vi "DoStuff.vi"(0 "Subnet in":refnum<class "Subnet.lvclass">, 9 "Steps":i32) -> (4 "Subnet out":refnum<class "Subnet.lvclass">, 6 "BroadcastCounter":u8, 8 "ValidCRC":i32, 10 "InvalidCRC":i32, 13 "CRCIssues":T1[](array[typedef]) {"Data" format="%02x"}, 14 "Messages":i32, 15 "error out":errorcluster)   [LabVIEW 2016]
uses:
  Subnet/Subnet.lvclass
  Common_RT_Modbus/DataTypes/RxFrame.ctl
  Subnet/Subnet.lvclass/Subnet.ctl
  Common_RT_HPILC/HPILC/HPILC.lvclass/HPILC.ctl
  Common_RT_HPILC/HPILC/HPILC.lvclass
  Common_RT_Modbus/RTModbus.lvlib
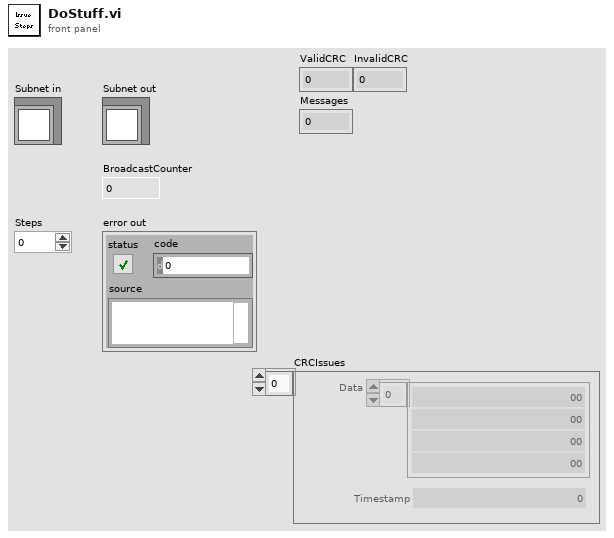
[diagram p1: front panel]
types:
  T1 = typedef "RTModbus.lvlib/RxFrame.ctl" = cluster{"Data":u8[], "Timestamp":u64}
  T2 = typedef "SubnetData.ctl" = cluster{"SubnetConstants":T3, "SubnetCommand":T6, "SubnetTelemetry":T7}
  T3 = typedef "SubnetConstants.ctl" = cluster{"Modbus":refnum<class "IModbus.lvclass">, "HPs":refnum<class "HPILC.lvclass">[], "AddressToActuator":T4[], "MTs":refnum<class "MTILC.lvclass">[], "MDs":refnum<class "MDILC.lvclass">[], "MIs":refnum<class "MIILC.lvclass">[]}
  T4 = typedef "ILCIndexData.ctl" = cluster{"ILCTypes":T5, "Index":i32}
  T5 = typedef "ILCTypes.ctl" = enum16{"Undefined", "SAA", "DAA", "HP", "MT", "MD", "MI"}
  T6 = typedef "SubnetCommand.ctl" = cluster{"BroadcastCounter":u8}
  T7 = typedef "SubnetTelemetry.ctl" = cluster{"BytesTransmitted":u32, "FramesTransmitted":u32, "BytesReceived":u32, "FramesReceived":u32, "TxInternalFIFOOverflow":bool, "InvalidInstruction":bool, "WaitForRxFrameTimeout":bool, "StartBitError":bool, "StopBitError":bool, "RxDataFIFOOverflow":bool}
  T8 = typedef "RTHPILC.lvlib/HPData.ctl" = cluster{"Constants":T9, "Command":T10, "Telemetry":T11, "Responses":T12, "Timings":T14}
  T9 = typedef "RTHPILC.lvlib/HPConstants.ctl" = cluster{"ID":i16, "ReferencePosition":i32}
  T10 = typedef "RTHPILC.lvlib/HPCommand.ctl" = cluster{"Steps":i8}
  T11 = typedef "RTHPILC.lvlib/HPTelemetry.ctl" = cluster{"ILCFault":bool, "LimitSwitchCWOperated":bool, "LimitSwitchCCWOperated":bool, "BroadcastCounter":u8, "SSIEncoderValue":i32, "LoadCellForce":sgl}
  T12 = typedef "RTHPILC.lvlib/HPResponses.ctl" = cluster{"StepMotor":T13, "ForceAndStatus":T13}
  T13 = typedef "RTModbus.lvlib/ExceptionCodes.ctl" = u16
  T14 = typedef "RTHPILC.lvlib/HPTimings.ctl" = cluster{"BroadcastStepMotor":u32, "ForceAndStatus":u32, "FreezeSensorValues":u32, "StepMotor":u32}
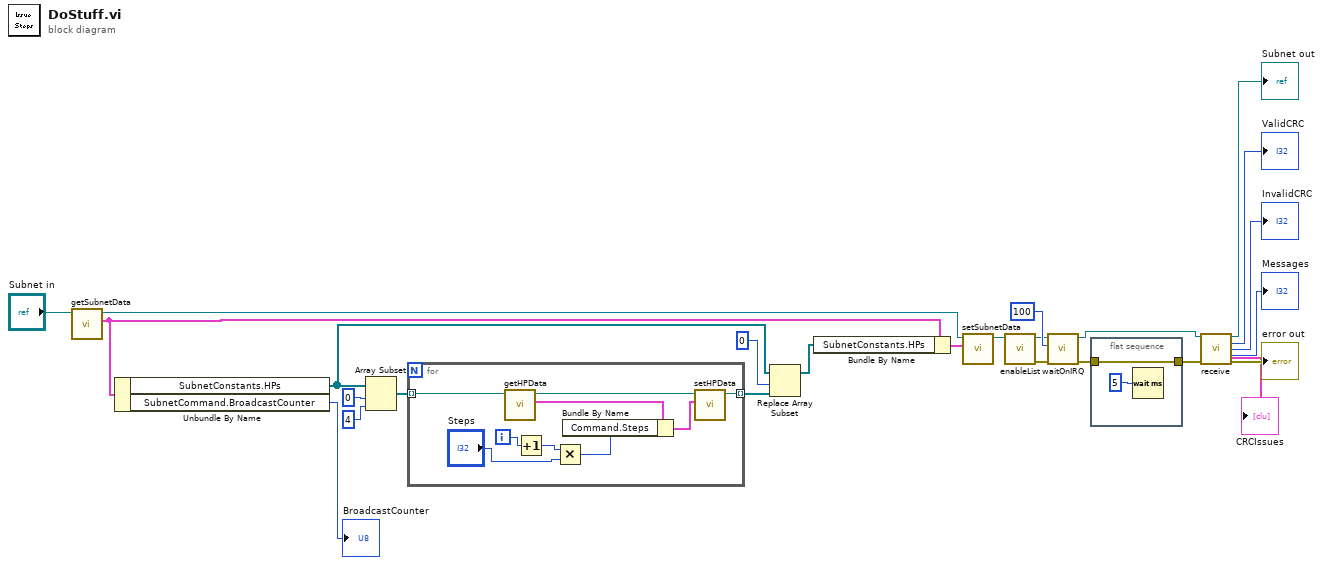
[diagram p0: block diagram]
diagram:
  n1 = call "getSubnetData.vi"("Subnet in"="Subnet in") -> ("SubnetData"=w16:T2, "Subnet out"=w18:refnum<class "Subnet.lvclass">)  [unwired: 9 in]
  n2 = Unbundle By Name(w16) -> ("SubnetConstants.HPs"=w10:refnum<class "HPILC.lvclass">[], "SubnetCommand.BroadcastCounter"=→"BroadcastCounter":u8)
  n3 = Array Subset(array=w10, index=0, length=4) -> (w11:refnum<class "HPILC.lvclass">[])
  n4 = for {
    tunnel: w11 -> [w31] mode=indexing
    tunnel: [w30] -> w8 mode=indexing
    i -> [w29]
    n5 = call "getHPData.vi"("HPILC in"=w31) -> ("HPData"=w34:T8, "HPILC out"=w32:refnum<class "HPILC.lvclass">)  [unwired: 9 in]
    n6 = Increment(x=w29) -> (x+1=w28:i32)
    n7 = Multiply(x=w28, y="Steps") -> (x*y=w26:i32)
    n8 = Bundle By Name(cluster=w34, "Command.Steps"=w26) -> (w33:T8)
    n9 = call "setHPData.vi"("HPData"=w33, "HPILC in"=w32) -> ("HPILC out"=w30:refnum<class "HPILC.lvclass">)  [unwired: 9 in]
  }
  n10 = Replace Array Subset(array=w10, new element=w8, index=0) -> (w7:refnum<class "HPILC.lvclass">[])
  n11 = Bundle By Name(cluster=w16, "SubnetConstants.HPs"=w7) -> (w17:T2)
  n12 = call "setSubnetData.vi"("SubnetData"=w17, "Subnet in"=w18) -> ("Subnet out"=w19:refnum<class "Subnet.lvclass">)  [unwired: 9 in]
  n13 = call-dynamic "enableList.vi"("Subnet in"=w19) -> ("error out"=w20:errorcluster, "Subnet out"=w14:refnum<class "Subnet.lvclass">)  [unwired: 9 in]
  n14 = call-dynamic "waitOnIRQ.vi"("error in (no error)"=w20, "Timeout (ms)"=100, "Subnet in"=w14) -> ("error out"=w3:errorcluster, "Subnet out"=w21:refnum<class "Subnet.lvclass">)  [unwired: 7 in]
  n15 = flat-sequence {
    tunnel: w3 -> [w35]
    tunnel: [w35] -> w2
    frame #0 {
      n16 = Wait (ms)(milliseconds to wait=u32 5) -> ()  [unwired: 1 out]
    }
  }
  n17 = call-dynamic "receive.vi"("Subnet in"=w21, "error in (no error)"=w2) -> ("Subnet out"=→"Subnet out":refnum<class "Subnet.lvclass">, "ValidCRC"=→"ValidCRC":i32, "InvalidCRC"=→"InvalidCRC":i32, "Messages"=→"Messages":i32, "CRCIssues"=→"CRCIssues":T1[], "error out"=→"error out":errorcluster)  [unwired: 8 in]
